vi "oa_TV Extract Geometric Imperfection (Analog Tacho NChan).vi"(0 "analog tacho signal":waveform(dbl)[](array[waveform]), 2 "missing pulses? (no:F)":bool[](array[boolean]), 3 "reset? (F)":bool, 5 "threshold (auto)":dbl[](array[numeric]), 7 "pulse/revolution":i32[](array[numeric]), 9 "hysteresis(0)":dbl[](array[numeric]), 11 "error in (no error)":errorcluster, 12 "pulse width (2)":i32[](array[numeric]), 14 "slope (Rising)":u16[](array[ring]) items=["Rising", "Falling"]) -> (4 "pulse positions":cluster{dbl[]}[](array[cluster]), 8 "revulotion":i32[](array[numeric]), 10 "revulotion index":i32[](array[numeric]), 15 "error out":errorcluster)   [LabVIEW 2017, in "SoundVib_Torsional.lvlib"]
uses:
  <vilib>/addons/Sound and Vibration/Order Analysis/Torsional Vibration/SoundVib_Torsional.lvlib
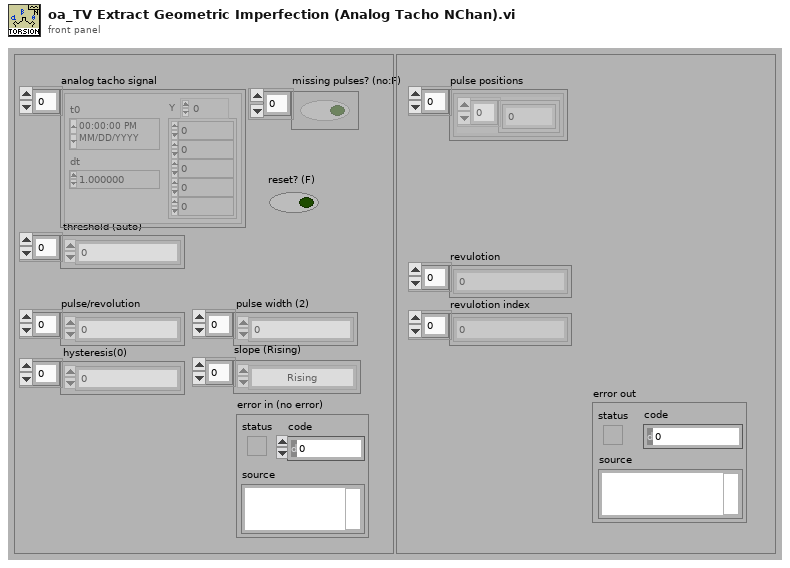
[diagram p1: front panel]
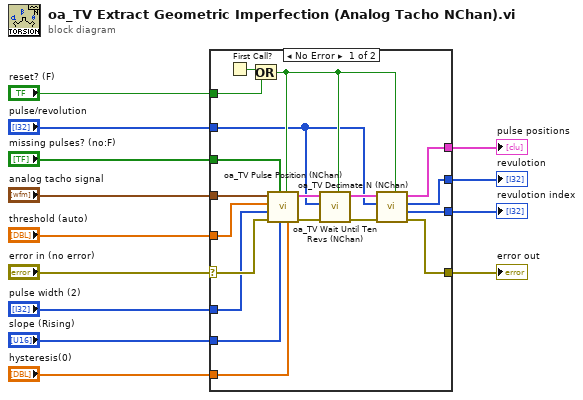
[diagram p0: block diagram]
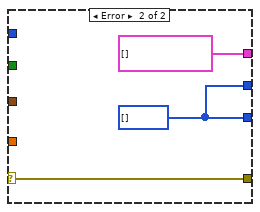
[diagram p2: hidden frame]
diagram:
  n1 = case shown="No Error" "error in (no error)" {
    selector: "error in (no error)" -> [w30 w35]
    tunnel: "analog tacho signal" -> [w28 _]
    tunnel: [w29 cluster{dbl[]}[] [] ("pulse positions")] -> w6
    tunnel: [w32 w33] -> w5
    tunnel: [w14 w35] -> w12
    tunnel: "threshold (auto)" -> [w21 _]
    tunnel: "pulse/revolution" -> [w17 _]
    tunnel: "pulse width (2)" -> [w19 _]
    tunnel: "slope (Rising)" -> [w20 _]
    tunnel: "hysteresis(0)" -> [w27 _]
    tunnel: "missing pulses? (no:F)" -> [w18 _]
    tunnel: "reset? (F)" -> [w16 _]
    tunnel: [w15 w33] -> w1
    frame No Error {
      n2 = First Call?() -> (First Call?: T/F=w31:bool)
      n3 = Or(x=w31, y=w16) -> (x .or. y?=w22:bool)
      n4 = call <vilib>:"oa_TV Pulse Position (NChan).vi"("hysteresis(0)"=w27, "reset? (F)"=w22, "slope (Rising)"=w20, "missing pulses? (no:F)"=w18, "error in (no error)"=w30, "pulse width (2)"=w19, "threshold (auto)"=w21, "analog tacho signal"=w28) -> ("error out"=w25:errorcluster, "pulse position [s]"=w26:cluster{dbl[]}[])  [unwired: 1 in, 1 out]
      n5 = call <vilib>:"oa_TV Wait Until Ten Revs (NChan).vi"("reset? (F)"=w22, "error in (no error)"=w25, "pulse/revolution"=w17, "pulse position [s]"=w26) -> ("error out"=w23:errorcluster, "pulse positions"=w24:cluster{dbl[]}[])  [unwired: 6 in]
      n6 = call <vilib>:"oa_TV Decimate N (NChan).vi"("reset? (F)"=w22, "error in (no error)"=w23, "pulse/revolution"=w17, "pulse position [s]"=w24) -> ("error out"=w14:errorcluster, "revulotion index"=w32:i32[], "revulotion"=w15:i32[], "pulse positions"=w29:cluster{dbl[]}[])  [unwired: 4 in]
    }
    frame Error {
      w33 = i32[] [] ("revulotion index")
    }
  }
  "error out" <- w12
  "pulse positions" <- w6
  "revulotion index" <- w5
  "revulotion" <- w1
